vi "Table.vi"(8 "error in":errorcluster, 11 "Loop Data In":T1={"VI Refnum"=refnum, "Timeout"=-1, "Code Data"=[], "Buffer Data"={"Connection ID"=refnum}, "Timer"=4294967295, "Image"=refnum}) -> (0 "error out":errorcluster, 2 "Table":string[][](array[string]), 3 "Loop Data Out":T1={"VI Refnum"=refnum, "Timeout"=-1, "Code Data"=[], "Buffer Data"={"Connection ID"=refnum}, "Timer"=4294967295, "Image"=refnum})   [LabVIEW 2016]
uses:
  Data Def/Loop Data.ctl
  Com/Matrix220/Data Def/Com_Matrix220_Buffer Data.ctl
  <vilib>/vision/Image Controls.llb/IMAQ Image.ctl
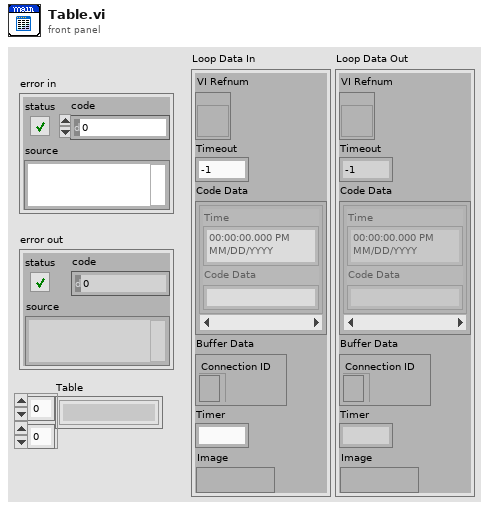
[diagram p1: front panel]
types:
  T1 = typedef "Loop Data.ctl" = cluster{"VI Refnum":refnum<vi>, "Timeout":i32, "Code Data":cluster{"Time":timestamp, "Code Data":string}[], "Buffer Data":T2, "Timer":u32, "Image":T3}
  T2 = typedef "Com_Matrix220_Buffer Data.ctl" = cluster{"Connection ID":refnum<k5>}
  T3 = typedef "IMAQ Image.ctl" = refnum<image>
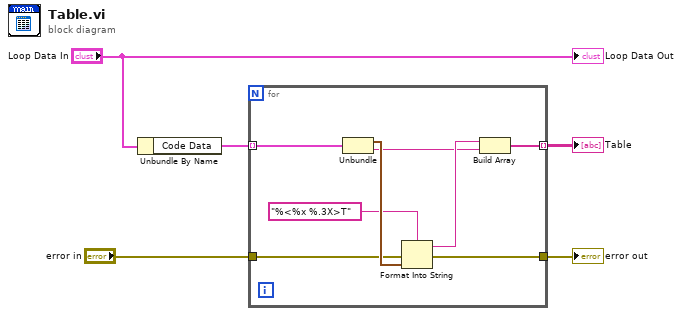
[diagram p0: block diagram]
diagram:
  n1 = Unbundle By Name("Loop Data In") -> ("Code Data"=w5:cluster{"Time":timestamp, "Code Data":string}[])
  n2 = for {
    tunnel: w5 -> [w13] mode=indexing
    tunnel: "error in" -> [w11]
    tunnel: [w7] -> w1
    tunnel: [w6] -> w3 mode=indexing
    n3 = Unbundle(w13) -> ("Time"=w12:timestamp, "Code Data"=w8:string)
    n4 = Format Into String(format string="%<%x %.3X>T", error in=w11, w12) -> (resulting string=w9:string, error out=w7:errorcluster)  [unwired: 1 in]
    n5 = Build Array(w9, w8) -> (w6:string[])
  }
  "error out" <- w1
  "Table" <- w3
  "Loop Data Out" <- "Loop Data In"
